vi "ParseJSONString.vi"(8 "error in (no error)":errorcluster, 11 "JSON string":string) -> (0 "error out":errorcluster, 3 "string":string)   [LabVIEW 2020]
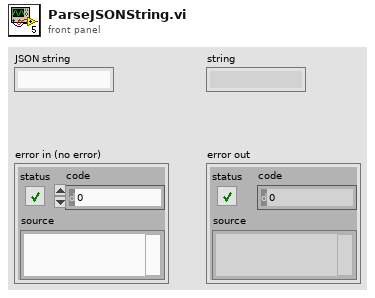
[diagram p1: front panel]
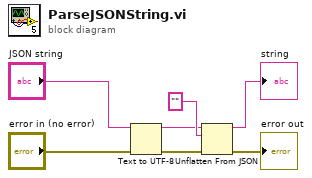
[diagram p0: block diagram]
diagram:
  n1 = Text to UTF-8(8:"error in (no error)", 11:"JSON string") -> (0:w5:errorcluster, 3:w1:string)  [unwired: 1 in]
  n2 = Unflatten From JSON(JSON string=w1, type and defaults="" ("whole match"), error in (no error)=w5) -> (value=→"string":string, error out=→"error out":errorcluster)  [unwired: 4 in]
